vi "poumiandata.vi"(0 "object in":refnum<class "212format_work.lvclass">, 1 "in":T2, 5 "error in (no error)":errorcluster) -> (14 "object out":refnum<class "212format_work.lvclass">, 15 "out":T1, 19 "error out":errorcluster)   [LabVIEW 2016, in "212format_work.lvclass"]
uses:
  212format_work.lvclass
  212format_work.lvclass/212format_work.ctl
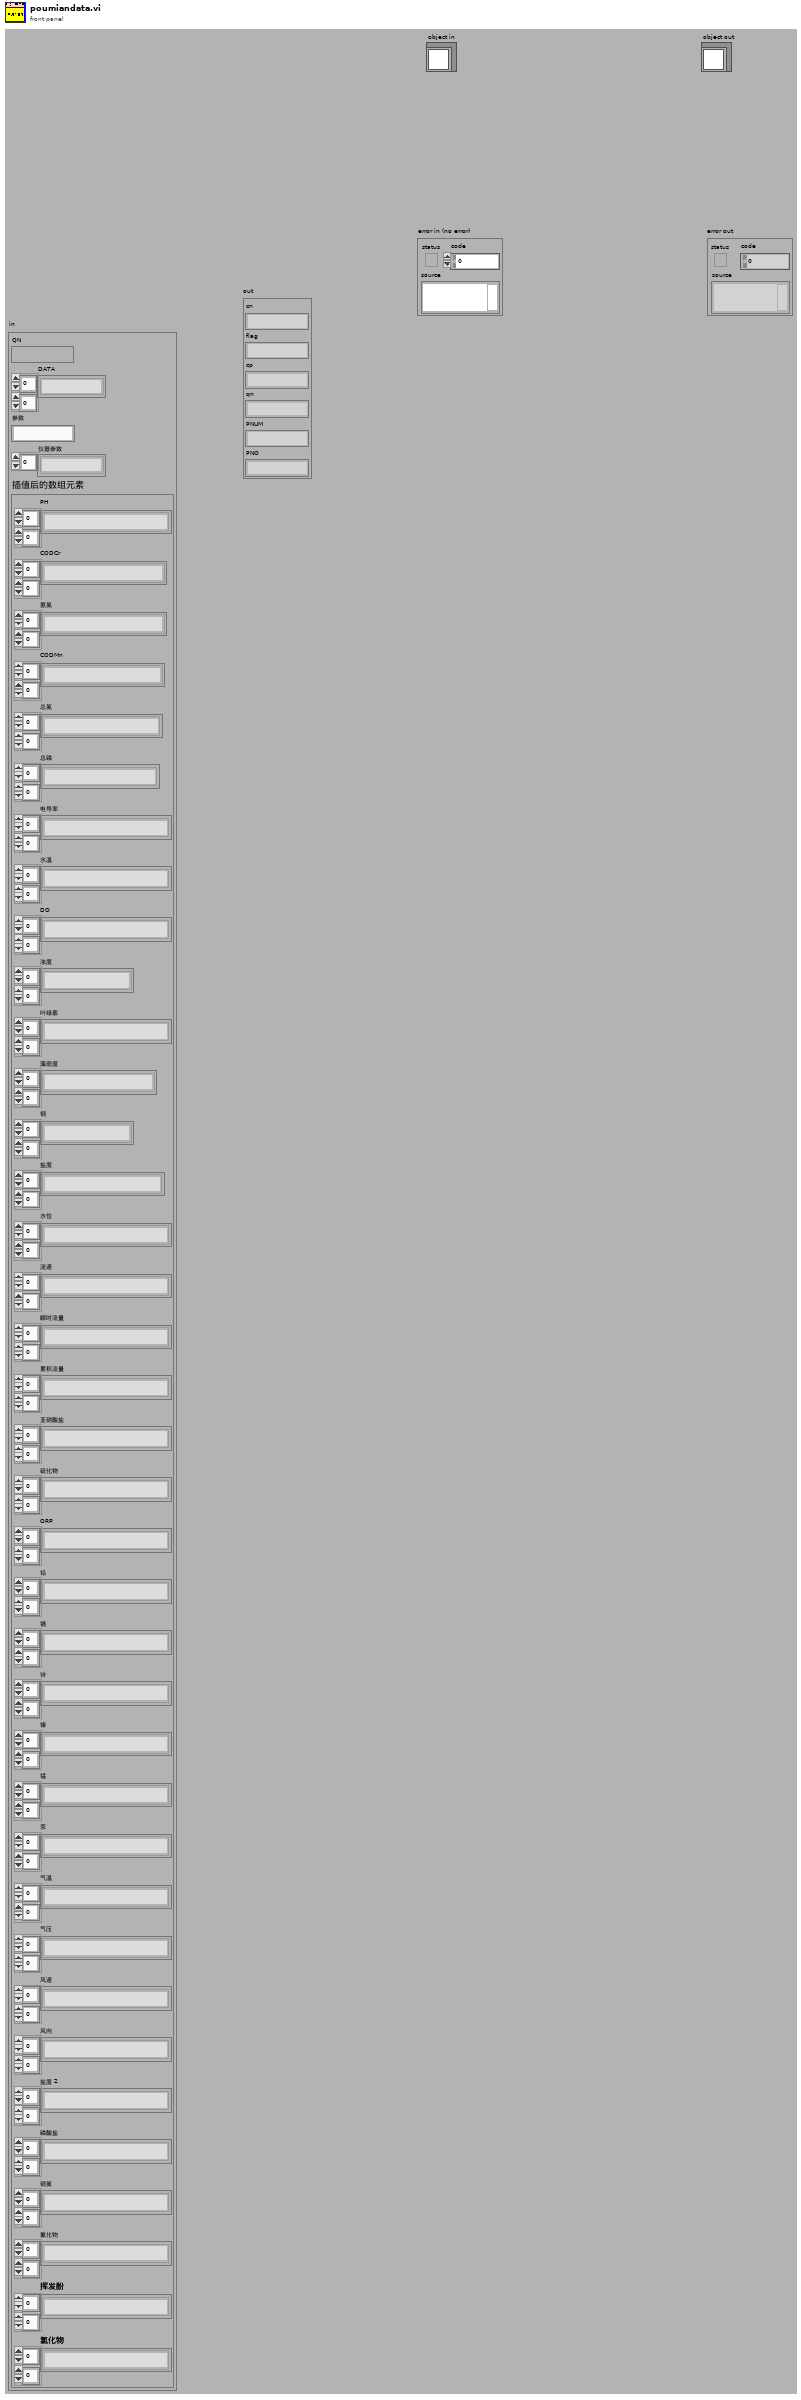
[diagram p1: front panel]
types:
  T1 = cluster{"cn":string, "flag":string, "cp":string, "qn":string, "PNUM":string, "PNO":string}
  T2 = cluster{"QN":string, "DATA":string[][], "参数":string, "仪器参数":string[], "插值后的数组元素":cluster{"PH":string[][], "CODCr":string[][], "氨氮":string[][], "CODMn":string[][], "总氮":string[][], "总磷":string[][], "电导率":string[][], "水温":string[][], "DO":string[][], "浊度":string[][], "叶绿素":string[][], "藻密度":string[][], "铜":string[][], "盐度":string[][], "水位":string[][], "流速":string[][], "瞬时流量":string[][], "累积流量":string[][], "亚硝酸盐":string[][], "硫化物":string[][], "ORP":string[][], "铅":string[][], "镉":string[][], "锌":string[][], "镍":string[][], "锰":string[][], "汞":string[][], "气温":string[][], "气压":string[][], "风速":string[][], "风向":string[][], "盐度 2":string[][], "磷酸盐":string[][], "硝氮":string[][], "氟化物":string[][], "挥发酚":string[][], "氯化物":string[][]}}
  T3 = enum16{"formattime", "formatminute", "formathour"}
  T4 = typedef "212format_work.lvclass/interdata控件.ctl" = cluster{"数据发送协议":enum16{"2005-212协议", "2017-212协议"}, "枚举":enum16{"返回请求应答", "上传数据", "返回执行结果"}, "系统编码ST":string, "主动上报数据中":bool, "数据组合发送":bool, "地表水/污染源":bool, "应用环境":enum16{"STD", "GB212"}}
  T5 = typedef "212format_work.lvclass/data控件.ctl" = cluster{"选择发送的参数":string, "插值后的数组元素":cluster{"PH":string[][], "CODCr":string[][], "氨氮":string[][], "CODMn":string[][], "总氮":string[][], "总磷":string[][], "电导率":string[][], "水温":string[][], "DO":string[][], "浊度":string[][], "叶绿素":string[][], "藻密度":string[][], "铜":string[][], "盐度":string[][], "水位":string[][], "流速":string[][], "瞬时流量":string[][], "累积流量":string[][], "亚硝酸盐":string[][], "硫化物":string[][], "ORP":string[][], "铅":string[][], "镉":string[][], "锌":string[][], "镍":string[][], "锰":string[][], "汞":string[][], "气温":string[][], "气压":string[][], "风速":string[][], "风向":string[][], "盐度 2":string[][], "磷酸盐":string[][], "硝氮":string[][], "氟化物":string[][], "挥发酚":string[][], "氯化物":string[][]}, "register values":u16[], "columns输出":string[], "环境参数":string[][], "仪器编码":string, "实时数据发送间隔":u32, "实时数据参数":string, "参数系数簇":cluster{"CODMn":dbl, "CODCr":dbl, "DO":dbl, "铜":dbl, "PH":dbl, "氨氮":dbl, "比电导率":dbl, "水温":dbl, "COD":dbl, "浊度":dbl, "总氮":dbl, "总磷":dbl, "叶绿素a":dbl, "藻密度":dbl, "水位":dbl, "流速":dbl, "瞬时流量":dbl, "累积流量":dbl, "亚硝酸盐":dbl, "硫化物":dbl, "ORP":dbl, "铅":dbl, "镉":dbl, "锌":dbl, "镍":dbl, "锰":dbl, "汞":dbl, "气温":dbl, "气压":dbl, "风速":dbl, "风向":dbl, "盐度":dbl, "磷酸盐":dbl, "硝氮":dbl, "氟化物":dbl, "挥发酚":dbl, "氯化物":dbl}, "因子编码簇":cluster{"CODMn":string, "CODCr":string, "DO":string, "铜":string, "PH":string, "氨氮":string, "比电导率":string, "水温":string, "COD":string, "浊度":string, "总氮":string, "总磷":string, "叶绿素a":string, "藻密度":string, "水位":string, "流速":string, "瞬时流量":string, "累积流量":string, "亚硝酸盐":string, "硫化物":string, "ORP":string, "铅":string, "镉":string, "锌":string, "镍":string, "锰":string, "汞":string, "气温":string, "气压":string, "风速":string, "风向":string, "盐度":string, "磷酸盐":string, "硝氮":string, "氟化物":string, "挥发酚":string, "氯化物":string}, "小时数据发送次数":i32, "读取试剂余量的值":u16[], "参数编码":string, "数据数组大小":i32, "总包数":i32, "当前包号":i32, "columns":string[], "剖面多参数":string[][], "分包标准":i32}
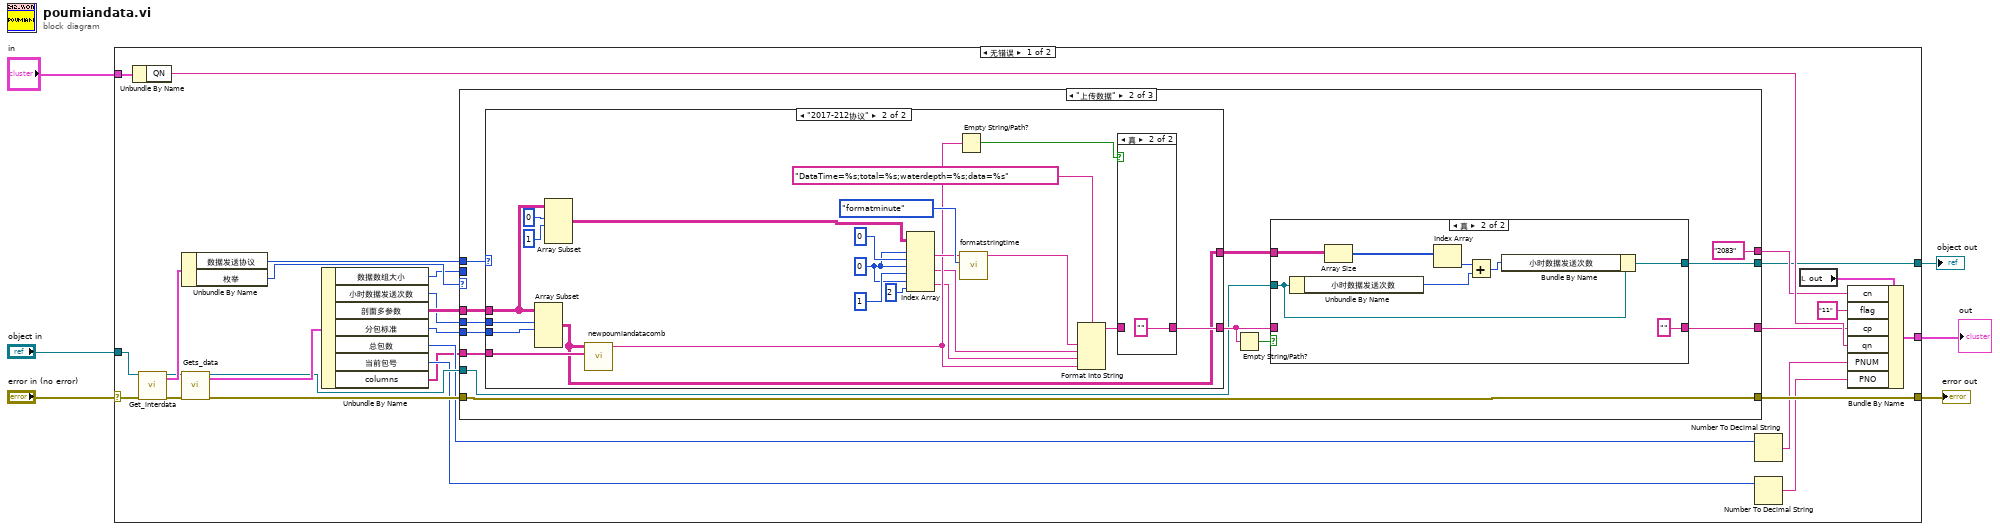
[diagram p0: block diagram]
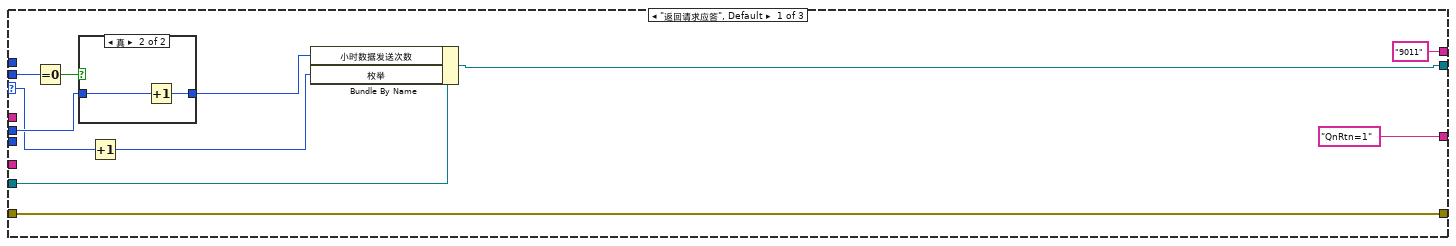
[diagram p2: hidden frame]
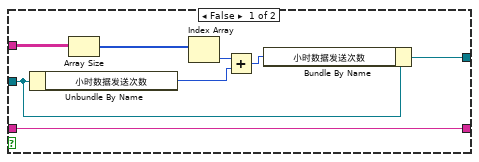
[diagram p4: hidden frame]
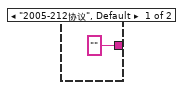
[diagram p5: hidden frame]
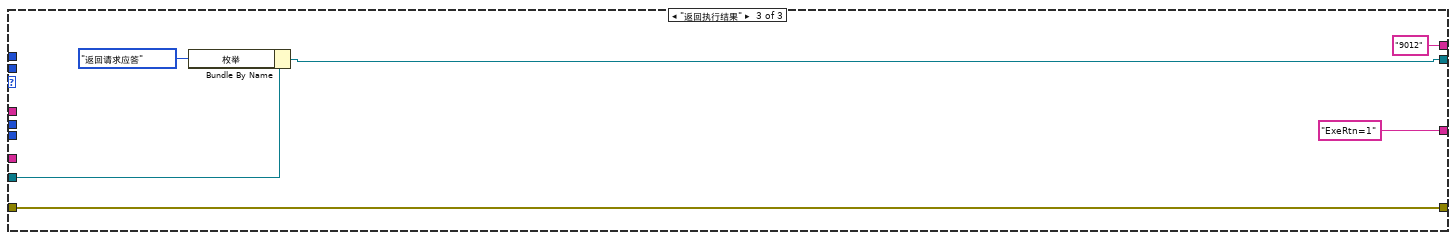
[diagram p7: hidden frame]
diagram:
  n1 = case shown="无错误" "error in (no error)" {
    selector: "error in (no error)" -> [w19 w110]
    tunnel: [w17 w110] -> w5
    tunnel: [w18 w109] -> w3
    tunnel: "object in" -> [w20 w109]
    tunnel: [w16 _] -> w2
    tunnel: "in" -> [w15 _]
    frame No Error {
      n2 = Unbundle By Name(w15) -> ("QN"=w33:string)
      n3 = call-dynamic "Get_interdata.vi"("object in"=w20, "error in (no error)"=w19) -> ("object out"=w27:refnum<class "212format_work.lvclass">, "interdata"=w29:T4, "error out"=w26:errorcluster)  [unwired: 15 in]
      n4 = Unbundle By Name(w29) -> ("数据发送协议"=w10:enum16{"2005-212协议", "2017-212协议"}, "枚举"=w28:enum16{"返回请求应答", "上传数据", "返回执行结果"})
      n5 = call-dynamic "Gets_data.vi"("object in"=w27, "error in (no error)"=w26) -> ("object out"=w22:refnum<class "212format_work.lvclass">, "data"=w25:T5, "error out"=w21:errorcluster)  [unwired: 15 in]
      n6 = Unbundle By Name(w25) -> ("数据数组大小"=w7:i32, "小时数据发送次数"=w23:i32, "剖面多参数"=w24:string[][], "分包标准"=w9:i32, "总包数"=w14:i32, "当前包号"=w13:i32, "columns"=w8:string[])
      n7 = case shown="\"上传数据\"" w28 {
        selector: w28 -> [w39 _ _]
        tunnel: ["9011" ("CN") "2083" ("CN") "9012" ("CN")] -> w32
        tunnel: ["QnRtn=1" w49 "ExeRtn=1"] -> w30
        tunnel: w22 -> [w43 w51 w106]
        tunnel: w24 -> [_ w58 _]
        tunnel: w23 -> [w41 w60 _]
        tunnel: [w37 w50 w104] -> w18
        tunnel: w21 -> [w36 w55 w103]
        tunnel: [w36 w55 w103] -> w17
        tunnel: w10 -> [_ w59 _]
        tunnel: w9 -> [_ w57 _]
        tunnel: w8 -> [_ w56 _]
        tunnel: w7 -> [w35 _ _]
        frame "返回请求应答", Default {
          n8 = Equal To 0?(x=w35) -> (x = 0?=w42:bool)
          n9 = case shown="真" w42 {
            tunnel: w41 -> [w46 w48]
            tunnel: [w46 w47] -> w40
            frame False {
            }
            frame True {
              n10 = Increment(x=w48) -> (x+1=w47:i32)
            }
          }
          n11 = Increment(x=w39) -> (x+1=w38:enum16{"返回请求应答", "上传数据", "返回执行结果"})
          n12 = Bundle By Name(cluster=w43, "小时数据发送次数"=w40, "枚举"=w38) -> (w37:refnum<class "212format_work.lvclass">)
        }
        frame "上传数据" {
          n13 = case shown="\"2017-212协议\"" w59 {
            tunnel: w60 -> [_ w99]
            tunnel: ["" ("编码输出") w80] -> w53
            tunnel: w58 -> [_ w94]
            tunnel: w57 -> [_ w98]
            tunnel: w56 -> [_ w97]
            tunnel: [_ w79] -> w52
            frame "2005-212协议", Default {
            }
            frame "2017-212协议" {
              w90 = 0 ("索引 (行)")
              n14 = Array Subset(array=w94, index (row)=w99, length (row)=w98) -> (w79:string[][])  [unwired: 2 in]
              n15 = Array Subset(array=w94, index (row)=0 ("索引"), length (row)=1 ("长度")) -> (w89:string[][])  [unwired: 2 in]
              n16 = call "newpoumiandatacomb.vi"("columns"=w97, "剖面数据"=w79) -> ("结果字符串"=w84:string)  [unwired: 9 in]
              n17 = Index Array(array=w89, index (row) #1=w90, index (col) #1=0 ("索引 (行)"), index (row) #2=w90, index (col) #2=1 ("索引 (列)"), index (row) #3=w90, index (col) #3=2 ("索引 (列)")) -> (element #1=w88:string, element #2=w82:string, element #3=w83:string)
              n18 = Empty String/Path?(string/path=w84) -> (empty?=w86:bool)
              n19 = call "formatstringtime.vi"("枚举"=T3."formatminute", "字符串"=w88) -> ("result string"=w81:string)  [unwired: 9 in]
              n20 = Format Into String(format string="DataTime=%s;total=%s;waterdepth=%s;data=%s", w81, w82, w83, w84) -> (resulting string=w87:string)  [unwired: 2 in, 1 out]
              n21 = case shown="真" w86 {
                tunnel: [w101 ""] -> w80
                tunnel: w87 -> [w101 _]
                frame False {
                }
                frame True {
                }
              }
            }
          }
          n22 = Empty String/Path?(string/path=w53) -> (empty?=w54:bool)
          n23 = case shown="真" w54 {
            tunnel: [w69 ""] -> w49
            tunnel: w53 -> [w69 _]
            tunnel: w52 -> [w68 w75]
            tunnel: w51 -> [w65 w71]
            tunnel: [w62 w72] -> w50
            frame False {
              n24 = Unbundle By Name(w65) -> ("小时数据发送次数"=w64:i32)
              n25 = Array Size(array=w68) -> (size(s)=w67:i32[])
              n26 = Index Array(array=w67) -> (element=w66:i32)  [unwired: 1 in]
              n27 = Add(x=w66, y=w64) -> (x+y=w63:i32)
              n28 = Bundle By Name(cluster=w65, "小时数据发送次数"=w63) -> (w62:refnum<class "212format_work.lvclass">)
            }
            frame True {
              n29 = Unbundle By Name(w71) -> ("小时数据发送次数"=w70:i32)
              n30 = Array Size(array=w75) -> (size(s)=w76:i32[])
              n31 = Index Array(array=w76) -> (element=w73:i32)  [unwired: 1 in]
              n32 = Add(x=w73, y=w70) -> (x+y=w74:i32)
              n33 = Bundle By Name(cluster=w71, "小时数据发送次数"=w74) -> (w72:refnum<class "212format_work.lvclass">)
            }
          }
        }
        frame "返回执行结果" {
          n34 = Bundle By Name(cluster=w106, "枚举"=enum16{"返回请求应答", "上传数据", "返回执行结果"}."返回请求应答" ("interdata.枚举")) -> (w104:refnum<class "212format_work.lvclass">)
        }
      }
      n35 = Number To Decimal String(number=w14) -> (decimal integer string=w12:string)  [unwired: 1 in]
      n36 = Number To Decimal String(number=w13) -> (decimal integer string=w11:string)  [unwired: 1 in]
      n37 = local read "out"() -> (w34:T1)
      n38 = Bundle By Name(cluster=w34, "cn"=w32, "flag"="11" ("ST"), "cp"=w30, "qn"=w33, "PNUM"=w12, "PNO"=w11) -> (w16:T1)
    }
    frame Error {
    }
  }
  "error out" <- w5
  "object out" <- w3
  "out" <- w2
